vi "D_Datagrid in subpanel example.vi"() -> ()   [LabVIEW 2018, in "D Datagrid Library.lvlib"]
uses:
  D Datagrid Library.lvlib
  D_Datagrid example.vi
panel:
  in  "stop":bool
  # "Subpanels have a bug that do not let them\nproperly convert local coordinates to screen\ncoordinates. Thus, to work in a subpanel,\nyou have to manually give it the reference\nof the VI that owns the subpanel."
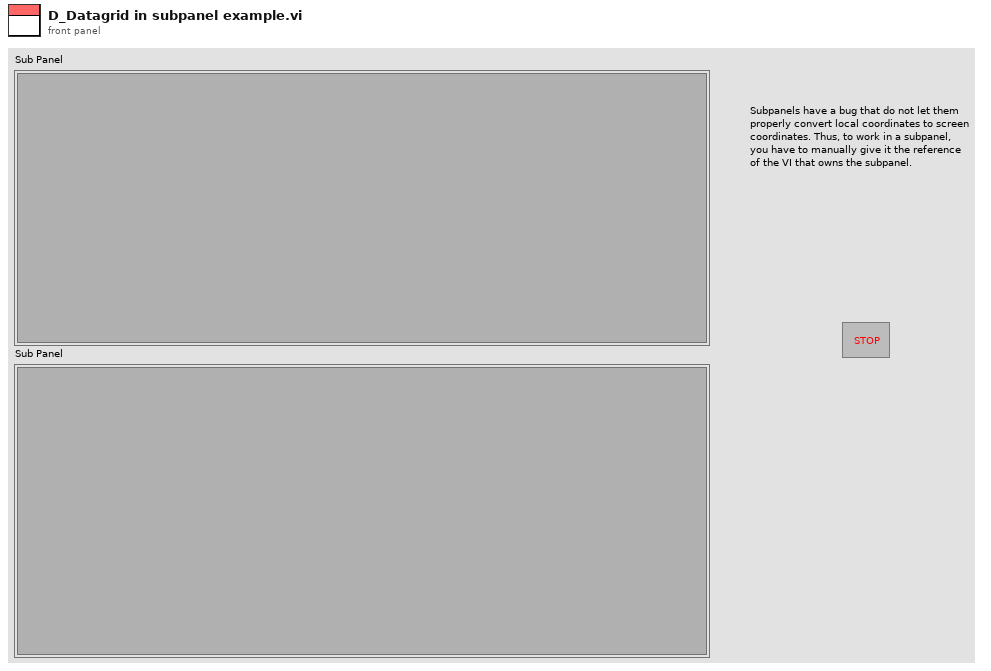
[diagram p1: front panel]
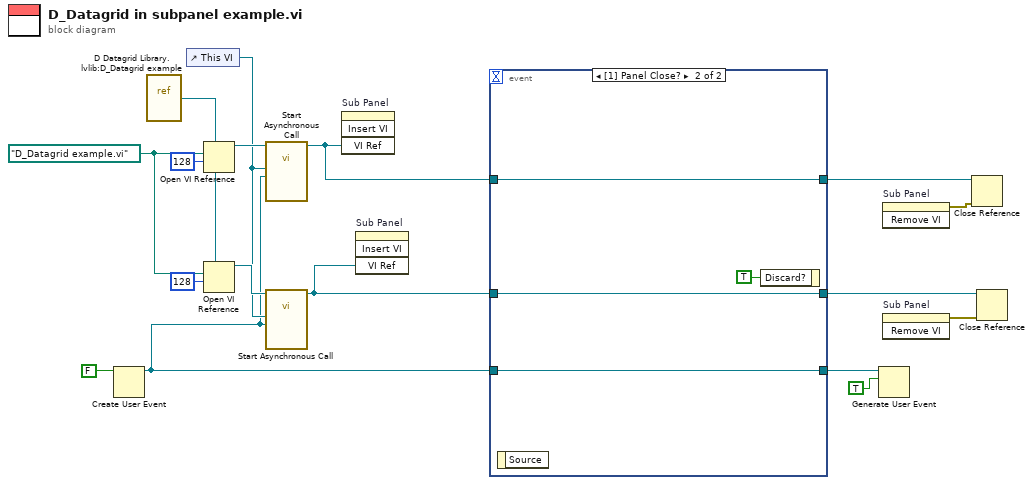
[diagram p0: block diagram]
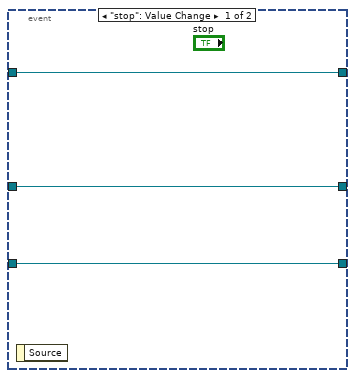
[diagram p2: hidden frame]
diagram:
  w15 = path "D_Datagrid example.vi" ("vi path")
  n1 = Create User Event(user event datatype=FALSE ("stop")) -> (user event=w4:refnum<user-event>)  [unwired: 1 in, 1 out]
  n2 = vi-ref "D Datagrid Library.lvlib:D_Datagrid example.vi"() -> (w14:refnum<vi>)
  n3 = control-ref of="This VI"() -> (w11:refnum<vi>)
  n4 = Open VI Reference(type specifier VI Refnum (for type only)=w14, vi path=w15, options=128) -> (vi reference=w13:refnum<vi>)  [unwired: 3 in, 1 out]
  n5 = Open VI Reference(type specifier VI Refnum (for type only)=w14, vi path=w15, options=128) -> (vi reference=w12:refnum<vi>)  [unwired: 3 in, 1 out]
  n6 = call-by-ref "Start Asynchronous Call"(reference=w13, "Remote stop event"=w4, "Owning VI"=w11) -> (reference out=w5:refnum<vi>)  [unwired: 11 in, 1 out]
  n7 = call-by-ref "Start Asynchronous Call"(reference=w12, "Remote stop event"=w4, "Owning VI"=w11) -> (reference out=w2:refnum<vi>)  [unwired: 11 in, 1 out]
  n8 = invoke on="Sub Panel" class="SubPnl" method="Insert VI"("VI Ref"=w5) -> ()  [unwired: 3 in, 4 out]
  n9 = invoke on="Sub Panel" class="SubPnl" method="Insert VI"("VI Ref"=w2) -> ()  [unwired: 3 in, 4 out]
  n10 = event shown="[1] Panel Close?" {
    selector: _ -> [_ _]
    dyn-events: _ -> [_ _]
    timeout: _ -> [_ _]
    tunnel: [w20 w23] -> w6
    tunnel: w5 -> [w20 w23]
    tunnel: [w19 w22] -> w3
    tunnel: w4 -> [w19 w22]
    tunnel: w2 -> [w18 w21]
    tunnel: [w18 w21] -> w1
    event "stop": Value Change {
      n11 = event-data() -> ()  [unwired: 1 in, 1 out]
    }
    event Panel Close? {
      n12 = event-data() -> ()  [unwired: 1 in, 1 out]
      n13 = event-data("Discard?"=TRUE) -> ()  [unwired: 1 in, 1 out]
    }
  }
  n14 = Generate User Event(user event=w3, event data cluster=TRUE ("event data")) -> ()  [unwired: 2 in, 2 out]
  n15 = invoke on="Sub Panel" class="SubPnl" method="Remove VI"() -> (error out=w8:errorcluster)  [unwired: 3 in, 2 out]
  n16 = invoke on="Sub Panel" class="SubPnl" method="Remove VI"() -> (error out=w9:errorcluster)  [unwired: 3 in, 2 out]
  n17 = Close Reference(reference=w6, error in (no error)=w8) -> ()  [unwired: 1 out]
  n18 = Close Reference(reference=w1, error in (no error)=w9) -> ()  [unwired: 1 out]
